vi "HDLC_send_frame.vi"(10 "data":u8[](array[numeric]), 11 "VISA resource name":refnum<visa-resource-name>) -> ()   [LabVIEW 2018]
uses:
  special_characters.ctl
panel:
  in  "crc":u16=65535 format="%x"
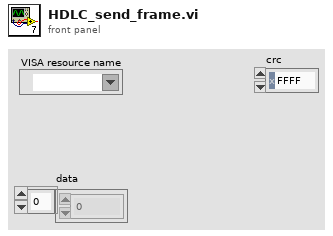
[diagram p1: front panel]
types:
  T1 = typedef "special_characters.ctl" = u8
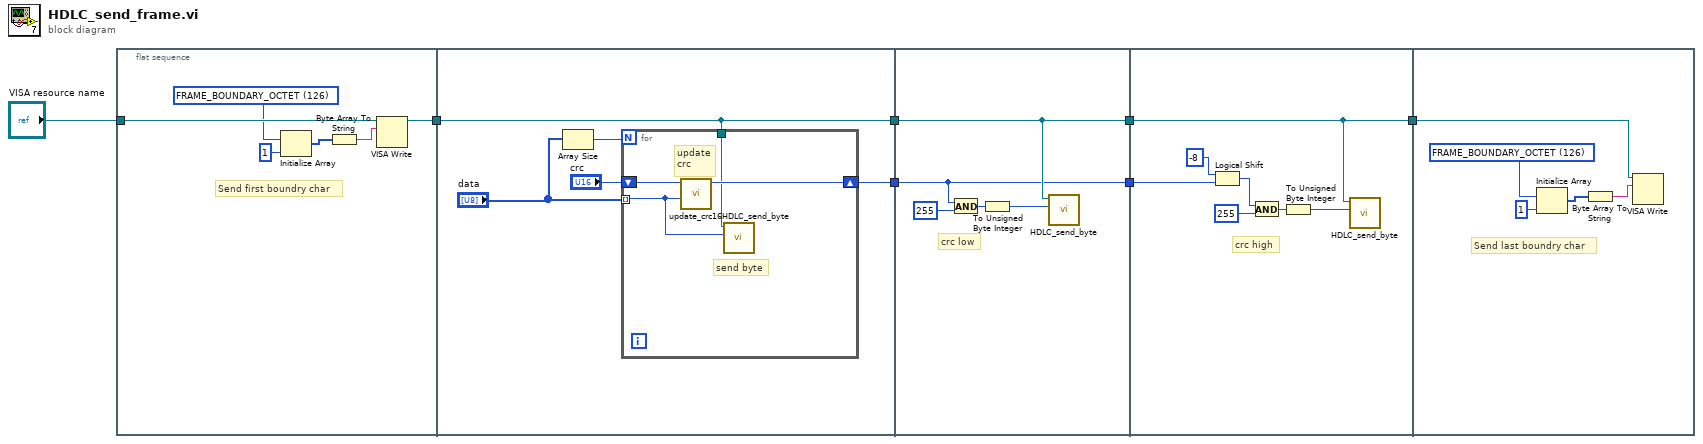
[diagram p0: block diagram]
diagram:
  n1 = flat-sequence {
    tunnel: "VISA resource name" -> [w13]
    tunnel: [w8] -> w6
    tunnel: w6 -> [w14]
    tunnel: [w14] -> w5
    tunnel: [w15] -> w4
    tunnel: w5 -> [w24]
    tunnel: w4 -> [w23]
    tunnel: [w24] -> w3
    tunnel: [w23] -> w2
    tunnel: w3 -> [w31]
    tunnel: w2 -> [w28]
    tunnel: [w31] -> w1
    tunnel: w1 -> [w35]
    frame #0 {
      w11 = T1 126 items=["FRAME_BOUNDARY_OCTET"=126, "CONTROL_ESCAPE_OCTET"=125, "INVERT_OCTET"=32] ("Ring")
      # "Send first boundry char"
      n2 = Initialize Array(w11, 1 ("dimension size")) -> (w9:T1[])
      n3 = Byte Array To String(unsigned byte array=w9) -> (string=w12:string)
      n4 = VISA Write(VISA resource name=w13, write buffer=w12) -> (VISA resource name out=w8:refnum<visa-resource-name>)  [unwired: 1 in, 2 out]
    }
    frame #1 {
      n5 = Array Size(array="data") -> (size(s)=w18:i32)
      n6 = for {
        N: w18 -> [_]
        tunnel: "data" -> [w19] mode=indexing
        shift-right: [w21] -> w15
        shift-left: "crc" -> [w22]
        tunnel: w14 -> [w20]
        # "update\ncrc"
        # "send byte"
        n7 = call "update_crc16.vi"("data"=w19, "crc"=w22) -> ("new_crc"=w21:u16)  [unwired: 9 in]
        n8 = call "HDLC_send_byte.vi"("byte"=w19, "VISA resource name"=w20) -> ()  [unwired: 10 in]
      }
    }
    frame #2 {
      # "crc low"
      n9 = And(x=w23, y=u16 255) -> (x .and. y?=w26:u16)
      n10 = To Unsigned Byte Integer(number=w26) -> (unsigned 8bit integer=w25:u8)
      n11 = call "HDLC_send_byte.vi"("byte"=w25, "VISA resource name"=w24) -> ()  [unwired: 10 in]
    }
    frame #3 {
      # "crc high"
      n12 = Logical Shift(y=i16 -8, x=w28) -> (x << y=w30:u16)
      n13 = And(x=w30, y=u16 255) -> (x .and. y?=w33:u16)
      n14 = To Unsigned Byte Integer(number=w33) -> (unsigned 8bit integer=w32:u8)
      n15 = call "HDLC_send_byte.vi"("byte"=w32, "VISA resource name"=w31) -> ()  [unwired: 10 in]
    }
    frame #4 {
      w38 = T1 126 items=["FRAME_BOUNDARY_OCTET"=126, "CONTROL_ESCAPE_OCTET"=125, "INVERT_OCTET"=32] ("Ring")
      # "Send last boundry char"
      n16 = Initialize Array(w38, 1 ("dimension size")) -> (w36:T1[])
      n17 = Byte Array To String(unsigned byte array=w36) -> (string=w39:string)
      n18 = VISA Write(VISA resource name=w35, write buffer=w39) -> ()  [unwired: 1 in, 3 out]
    }
  }
